vi "SetCellColor.vi"(5 "列":i32, 7 "行":i32, 8 "error":errorcluster caption="错误输入（无错误）", 9 "取消颜色设置":bool, 10 "颜色盒":u32(colorbox), 11 "Excel._Worksheet":refnum<k7>) -> (0 "error out":errorcluster caption="错误输出", 3 "Excel._Worksheet":refnum<k7>)   [LabVIEW 2014]
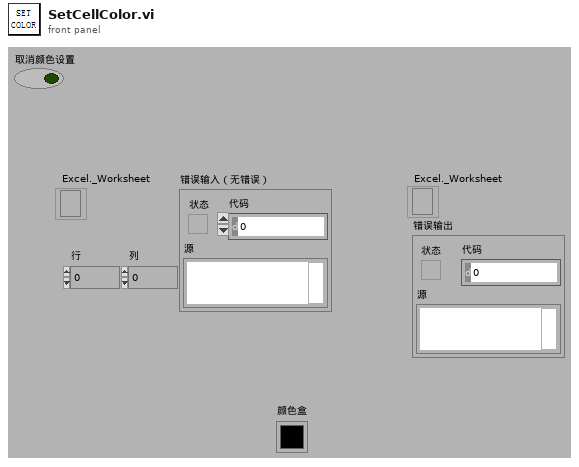
[diagram p1: front panel]
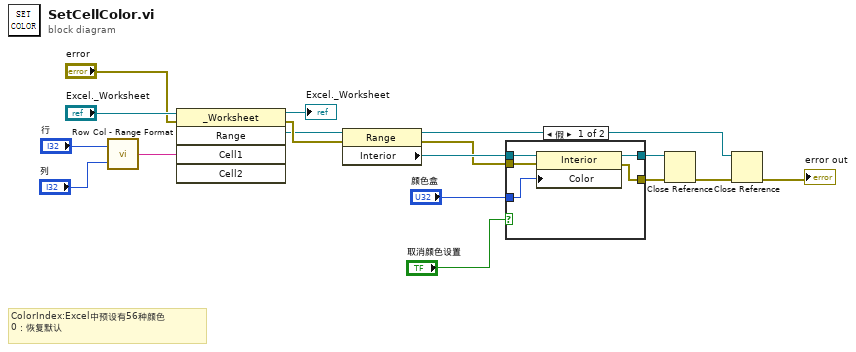
[diagram p0: block diagram]
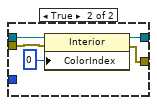
[diagram p2: hidden frame]
diagram:
  # "ColorIndex:Excel中预设有56种颜色\n0：恢复默认"
  n1 = call "Row Col - Range Format.vi"("Column"="列", "Row"="行") -> ("Output String"=w1:string)
  n2 = invoke class="_Worksheet" method="Range"(reference="Excel._Worksheet", error in="error", "Cell1"=w1) -> (reference out=→"Excel._Worksheet":refnum<k7>, error out=w13:errorcluster, "Range"=w11:refnum<k7>)  [unwired: 2 in, 2 out]
  n3 = property class="Range"(reference=w11, error in=w13) -> (reference out=w6:refnum<k7>, error out=w2:errorcluster, "Interior"=w10:refnum<k7>)
  n4 = case shown="假" "取消颜色设置" {
    tunnel: w10 -> [w22 w27]
    tunnel: [w21 w26] -> w9
    tunnel: [w20 w24] -> w8
    tunnel: "颜色盒" -> [w18 _]
    tunnel: w2 -> [w19 w23]
    frame False {
      n5 = property class="Interior"(reference=w22, error in=w19, "Color"=w18) -> (reference out=w21:refnum<k7>, error out=w20:errorcluster)
    }
    frame True {
      n6 = property class="Interior"(reference=w27, error in=w23, "ColorIndex"=0) -> (reference out=w26:refnum<k7>, error out=w24:errorcluster)
    }
  }
  n7 = Close Reference(reference=w9, error in (no error)=w8) -> (error out=w7:errorcluster)
  n8 = Close Reference(reference=w6, error in (no error)=w7) -> (error out=→"error out":errorcluster)
